vi "CTI_AOTF_StoreChannelFromGlobalVars.vi"(8 "error in":errorcluster) -> (0 "error out":errorcluster)   [LabVIEW 2011]
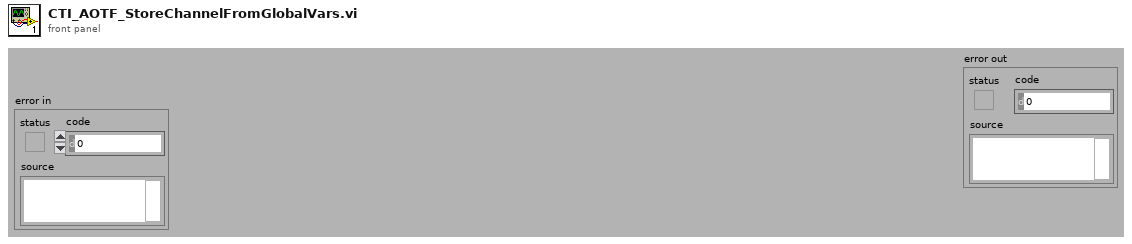
[diagram p1: front panel]
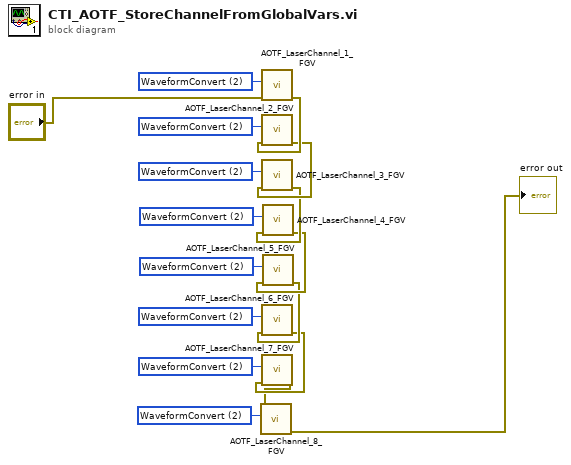
[diagram p0: block diagram]
diagram:
  w8 = u16 2 items=["Set", "Get", "WaveformConvert"] ("Set_Get")
  w9 = u16 2 items=["Set", "Get", "WaveformConvert"] ("Set_Get")
  w10 = u16 2 items=["Set", "Get", "WaveformConvert"] ("Set_Get")
  w11 = u16 2 items=["Set", "Get", "WaveformConvert"] ("Set_Get")
  w12 = u16 2 items=["Set", "Get", "WaveformConvert"] ("Set_Get")
  w13 = u16 2 items=["Set", "Get", "WaveformConvert"] ("Set_Get")
  w14 = u16 2 items=["Set", "Get", "WaveformConvert"] ("FGV_Control")
  w15 = u16 2 items=["Set", "Get", "WaveformConvert", ""] ("Set_Get")
  n1 = call "AOTF_LaserChannel_1_FGV.vi"("error in"="error in", "Set_Get"=w15) -> ("error out"=w7:errorcluster)  [unwired: 8 in, 1 out]
  n2 = call "AOTF_LaserChannel_2_FGV.vi"("error in"=w7, "FGV_Control"=w14) -> ("error out"=w6:errorcluster)  [unwired: 8 in, 1 out]
  n3 = call "AOTF_LaserChannel_3_FGV.vi"("error in"=w6, "Set_Get"=w13) -> ("error out"=w5:errorcluster)  [unwired: 8 in, 1 out]
  n4 = call "AOTF_LaserChannel_4_FGV.vi"("error in"=w5, "Set_Get"=w12) -> ("error out"=w4:errorcluster)  [unwired: 8 in, 1 out]
  n5 = call "AOTF_LaserChannel_5_FGV.vi"("error in"=w4, "Set_Get"=w11) -> ("error out"=w3:errorcluster)  [unwired: 8 in, 1 out]
  n6 = call "AOTF_LaserChannel_6_FGV.vi"("error in"=w3, "Set_Get"=w10) -> ("error out"=w2:errorcluster)  [unwired: 8 in, 1 out]
  n7 = call "AOTF_LaserChannel_7_FGV.vi"("error in"=w2, "Set_Get"=w9) -> ("error out"=w1:errorcluster)  [unwired: 8 in, 1 out]
  n8 = call "AOTF_LaserChannel_8_FGV.vi"("error in"=w1, "Set_Get"=w8) -> ("error out"=→"error out":errorcluster)  [unwired: 8 in, 1 out]
